vi "HexCenterFinder.vi"() -> ()   [LabVIEW 2019]
uses:
  <vilib>/userDefined/High Color/IMAQdx.ctl
  <vilib>/Analysis/baseanly.llb/Mean (DBL).vi
  <vilib>/vision/driver/NI_Vision_Acquisition_Software.lvlib
  <vilib>/Analysis/NI_AALPro.lvlib
  <vilib>/vision/NI_Vision_Development_Module.lvlib
  <vilib>/Analysis/NI_AALBase.lvlib
panel:
  in  "Component":enum16{"Baseplate", "PCB", "Sensor"}(ring)
  out "concatenated string":string
  out "AngleAvg(3sides)":dbl
  out "CircleBad":T1 {"Radius" format="%.2f"; "Center"."Y" format="%.2f"; "Center"."X" format="%.2f"}
  out "Circle0":T1 {"Radius" format="%.2f"; "Center"."Y" format="%.4f"; "Center"."X" format="%.4f"}
  out "Y 3":dbl
  out "X 3":dbl
  out "Array":dbl[][](array[numeric])
  out "meanY":dbl format="%0.3f"
  out "meanX":dbl format="%0.3f"
  out "Center5":cluster{"X":sgl, "Y":sgl} {"Y" format="%.2f"; "X" format="%.2f"}
  out "Center4":cluster{"X":sgl, "Y":sgl} {"Y" format="%.2f"; "X" format="%.2f"}
  out "Center3":cluster{"X":sgl, "Y":sgl} {"Y" format="%.2f"; "X" format="%.2f"}
  out "Center2":cluster{"X":sgl, "Y":sgl} {"Y" format="%.2f"; "X" format="%.2f"}
  out "Center1":cluster{"X":sgl, "Y":sgl} {"Y" format="%.2f"; "X" format="%.2f"}
  out "Center (3sides)":cluster{"X":sgl, "Y":sgl} {"Y" format="%.4f"; "X" format="%.4f"}
  out "2sides \nBisecting Line":T2 {"Point 2"."Y" format="%.2f"; "Point 2"."X" format="%.2f"; "Point 1"."Y" format="%.2f"; "Point 1"."X" format="%.2f"}
  out "Y 2":dbl
  out "X 2":dbl
  out "Y":dbl
  out "X":dbl
  in  "Ysides":dbl[](array[numeric])=[893.5593, 821.0074, 821.9544]
  in  "Zpos":dbl[](array[numeric])=[66.4386, 66.953, 66.7995, 66.9366, 66.95, 66.95]
  in  "Xsides":dbl[](array[numeric])=[286.53, 329.344, 411.6833, 453.028, 411.403, 328.577]
  in  "Sides to use":enum16{"2 sides", "3 sides", "6 sides"}(ring)=enum."3 sides"
  out "Image":T3(plugin-control)
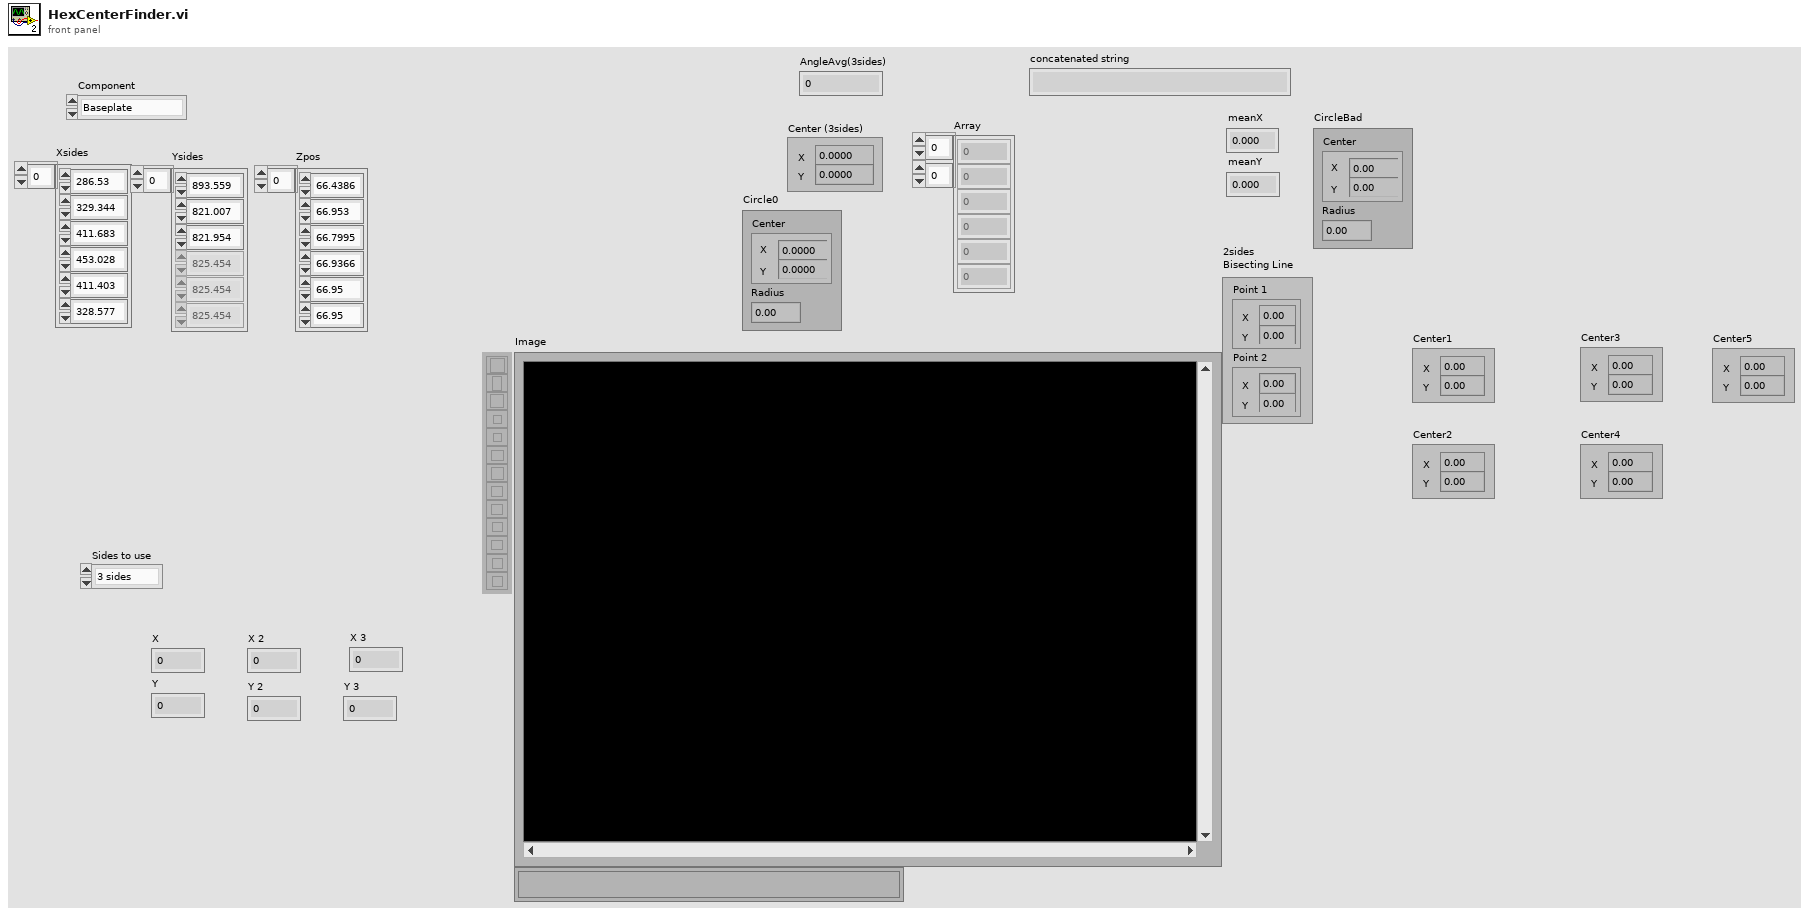
[diagram p1: front panel]
types:
  T1 = cluster{"Center":cluster{"X":sgl, "Y":sgl}, "Radius":dbl}
  T2 = cluster{"Point 1":cluster{"X":sgl, "Y":sgl}, "Point 2":cluster{"X":sgl, "Y":sgl}}
  T3 = typedef "IMAQ Image.ctl" = refnum<image>
  T4 = typedef "Image Type" = u32
  T5 = typedef "IMAQdx.ctl" = refnum<k21>
  T6 = typedef "IMAQ Line" = cluster{"Start X":i32, "Start Y":i32, "End X":i32, "End Y":i32}
  T7 = enum16{"open", "replace", "create", "open or create", "replace or create", "replace or create with confirmation"}
  T8 = cluster{cluster{"X":dbl, "Y":dbl}, cluster{"X":dbl, "Y":dbl}, cluster{"X":dbl, "Y":dbl}}
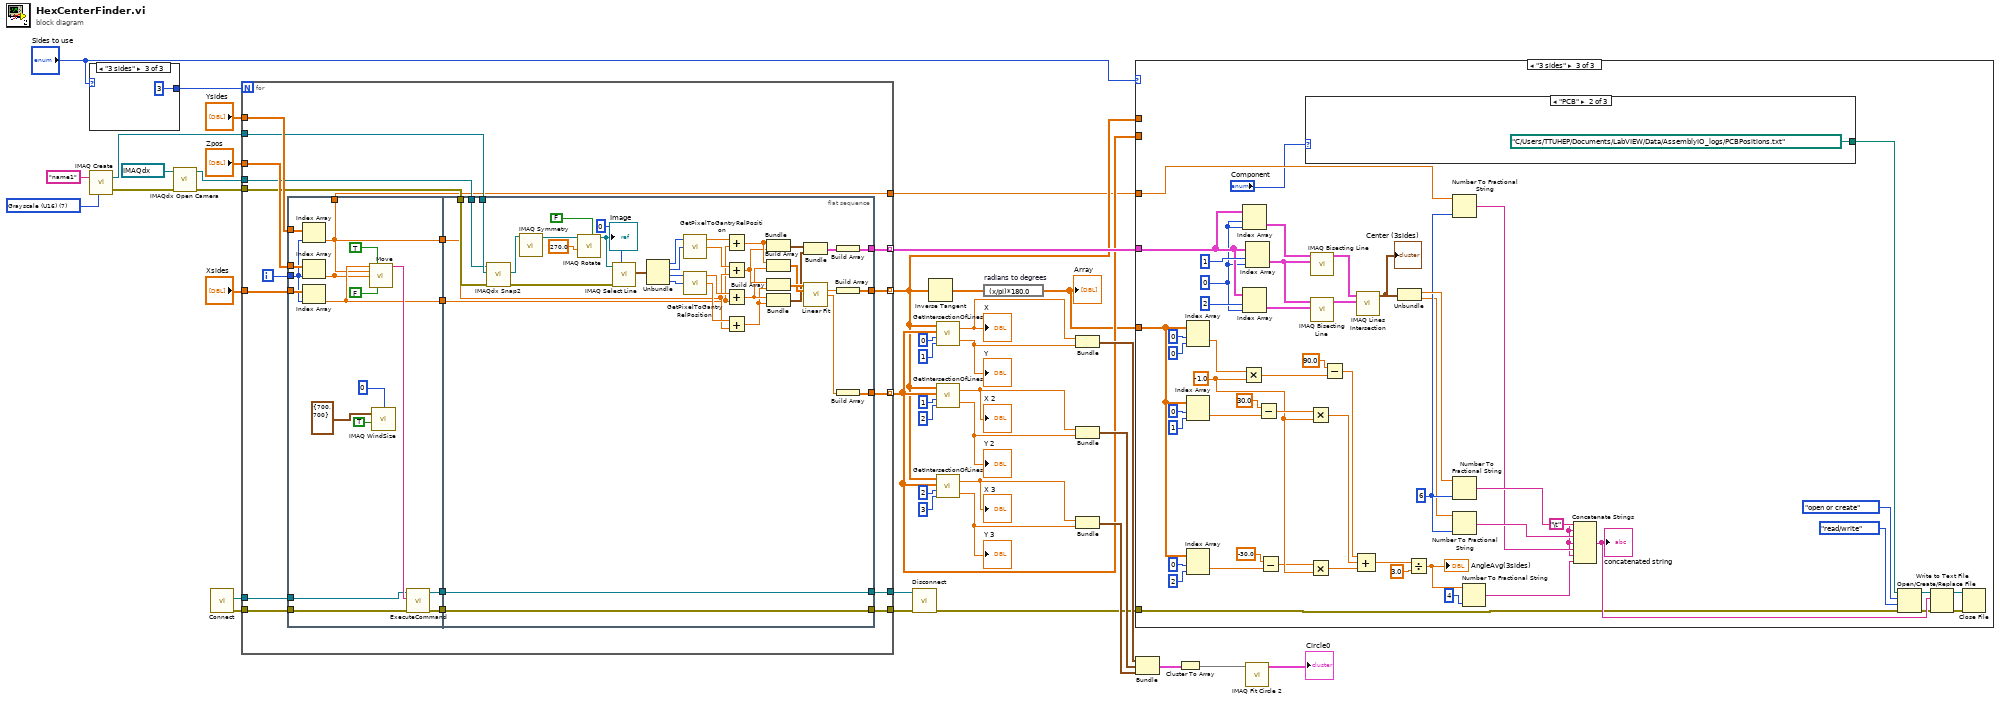
[diagram p0: block diagram]
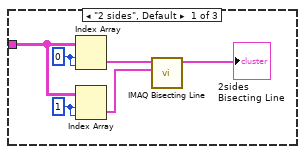
[diagram p2: hidden frame]
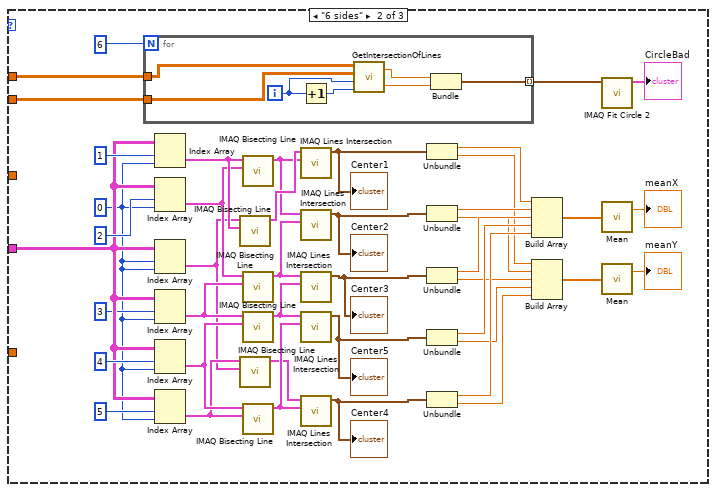
[diagram p3: hidden frame]
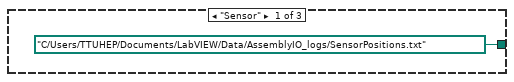
[diagram p4: hidden frame]
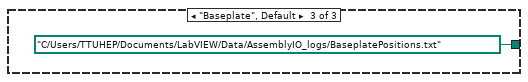
[diagram p5: hidden frame]
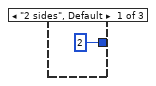
[diagram p6: hidden frame]
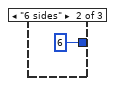
[diagram p7: hidden frame]
diagram:
  w38 = T4 7 items=["Grayscale (U8)", "Grayscale (I16)", "Grayscale (SGL)", "Complex (CSG)", "RGB (U32)", "HSL (U32)", "RGB (U64)", "Grayscale (U16)"] ("Image Type")
  n1 = case shown="\"3 sides\"" "Sides to use" {
    tunnel: [2 6 3] -> w37
    frame "2 sides", Default {
    }
    frame "6 sides" {
    }
    frame "3 sides" {
    }
  }
  n2 = call "IMAQ Create"("Image Name"="name1", "Image Type"=w38) -> ("New Image"=w29:T3, "error out"=w39:errorcluster)  [unwired: 3 in]
  n3 = call <vilib>:"IMAQdx Open Camera.vi"("error in"=w39, "Session In"=T5 "cam0") -> ("error out"=w30:errorcluster, "Session Out"=w28:T5)  [unwired: 8 in]
  n4 = call "Connect.vi"() -> ("error out"=w31:errorcluster, "controller"=w32:refnum<k24>)  [unwired: 10 in]
  n5 = for {
    N: w37 -> [_]
    tunnel: "Xsides" -> [w63]
    tunnel: "Ysides" -> [w62]
    tunnel: "Zpos" -> [w61]
    tunnel: [w59] -> w34
    tunnel: [w58] -> w33
    tunnel: w32 -> [w57]
    tunnel: w31 -> [w56]
    tunnel: w30 -> [w53]
    tunnel: w29 -> [w52]
    tunnel: w28 -> [w51]
    tunnel: [w48] -> w4 mode=indexing
    tunnel: [w47] -> w5 mode=indexing
    tunnel: [w46] -> w21 mode=indexing
    tunnel: [w45] -> w2
    i -> [w60]
    n6 = flat-sequence {
      tunnel: w63 -> [w80]
      tunnel: w62 -> [w79]
      tunnel: w61 -> [w78]
      tunnel: w60 -> [w77]
      tunnel: w57 -> [w71]
      tunnel: w56 -> [w70]
      tunnel: [w73] -> w55
      tunnel: [w72] -> w54
      tunnel: [w69] -> w50
      tunnel: [w68] -> w49
      tunnel: [w67] -> w45
      tunnel: [w116] -> w58
      tunnel: [w117] -> w59
      tunnel: w55 -> [w117]
      tunnel: w54 -> [w116]
      tunnel: w53 -> [w109]
      tunnel: w52 -> [w108]
      tunnel: w51 -> [w107]
      tunnel: w50 -> [w102]
      tunnel: w49 -> [w103]
      tunnel: [w100] -> w48
      tunnel: [w98] -> w47
      tunnel: [w82] -> w46
      frame #0 {
        n7 = Index Array(array=w79, index=w77) -> (element=w68:dbl)
        n8 = Index Array(array=w78, index=w77) -> (element=w67:dbl)
        n9 = Index Array(array=w80, index=w77) -> (element=w69:dbl)
        n10 = call "Move.vi"("X"=w69, "Absolute"=TRUE, "Y"=w68, "Z"=w67, "Move Z first"=FALSE) -> ("Position Gcode"=w74:string)  [unwired: 10 in]
        n11 = call "IMAQ WindSize"("Scrollbars? (N)"=TRUE, "Width & Height"=cluster{"Width":i32, "Height":i32} {"Width"=700, "Height"=700}, "Window Number"=0) -> ()  [unwired: 3 in, 3 out]
        n12 = call "ExecuteCommand.vi"("error in (no error)"=w70, "Command Code"=w74, "controller in"=w71) -> ("error out"=w73:errorcluster, "controller out"=w72:refnum<k24>)  [unwired: 6 in, 1 out]
      }
      frame #1 {
        n13 = call <vilib>:"IMAQdx Snap2.vi"("error in"=w109, "Image In"=w108, "Session In"=w107) -> ("error out"=w110:errorcluster, "Image Out"=w94:T3)  [unwired: 6 in, 1 out]
        n14 = call "IMAQ Symmetry"("Image Src"=w94) -> ("Image Dst Out"=w97:T3)  [unwired: 4 in, 1 out]
        n15 = call "IMAQ Rotate"("Maintain Size"=FALSE, "Angle (degrees)"=sgl 270.0, "Image Src"=w97) -> ("Image Dst Out"=w93:T3)  [unwired: 7 in, 1 out]
        "Image" <- w93
        n16 = call "IMAQ Select Line"("Window Number (0...15)"=0, "error in (no error)"=w110, "Image In"=w93) -> ("Line"=w111:T6)  [unwired: 5 in, 3 out]
        n17 = Unbundle(w111) -> ("Start X"=w112:i32, "Start Y"=w113:i32, "End X"=w114:i32, "End Y"=w115:i32)
        n18 = call "GetPixelToGantryRelPosition.vi"("PixelY"=w113, "PixelX"=w112) -> ("YmmRelGH"=w104:dbl, "XmmRelGH"=w90:dbl)  [unwired: 1 in, 1 out]
        n19 = call "GetPixelToGantryRelPosition.vi"("PixelY"=w115, "PixelX"=w114) -> ("YmmRelGH"=w105:dbl, "XmmRelGH"=w106:dbl)  [unwired: 1 in, 1 out]
        n20 = Add(x=w90, y=w102) -> (x+y=w89:dbl)
        n21 = Add(x=w104, y=w103) -> (x+y=w88:dbl)
        n22 = Add(x=w106, y=w102) -> (x+y=w87:dbl)
        n23 = Add(x=w105, y=w103) -> (x+y=w86:dbl)
        n24 = Bundle(w89, w88) -> (w85:cluster{dbl, dbl})  [unwired: 1 in]
        n25 = Build Array(w89, w87) -> (w91:dbl[])
        n26 = Build Array(w88, w86) -> (w92:dbl[])
        n27 = Bundle(w87, w86) -> (w84:cluster{dbl, dbl})  [unwired: 1 in]
        n28 = Bundle(w85, w84) -> (w83:cluster{cluster{dbl, dbl}, cluster{dbl, dbl}})  [unwired: 1 in]
        n29 = call <vilib>:"Linear Fit.vi"("Y"=w92, "X"=w91) -> ("slope"=w101:dbl, "intercept"=w99:dbl)  [unwired: 9 in, 3 out]
        n30 = Build Array(w83) -> (w82:cluster{cluster{dbl, dbl}, cluster{dbl, dbl}}[])
        n31 = Build Array(w101) -> (w100:dbl[])
        n32 = Build Array(w99) -> (w98:dbl[])
      }
    }
  }
  n33 = call "Disconnect.vi"("error in (no error)"=w34, "controller"=w33) -> ("error out"=w1:errorcluster)  [unwired: 9 in]
  n34 = Inverse Tangent(1:w4) -> (0:w27:dbl[][])
  n35 = call "GetIntersectionOfLines.vi"("Line1Idx"=1, "Line0Idx"=0, "InterceptArray"=w5, "SlopeArray"=w4) -> ("Y"=w16:dbl, "X"=w17:dbl)
  "X" <- w17
  "Y" <- w16
  n36 = call "GetIntersectionOfLines.vi"("Line1Idx"=2, "Line0Idx"=1, "InterceptArray"=w5, "SlopeArray"=w4) -> ("Y"=w14:dbl, "X"=w15:dbl)
  "X 2" <- w15
  "Y 2" <- w14
  n37 = call "GetIntersectionOfLines.vi"("Line1Idx"=3, "Line0Idx"=2, "InterceptArray"=w5, "SlopeArray"=w4) -> ("Y"=w12:dbl, "X"=w13:dbl)
  "X 3" <- w13
  "Y 3" <- w12
  n38 = expression code="(x/pi)*180.0" "radians to degrees"(w27) -> (w3:dbl[][])
  "Array" <- w3
  n39 = Bundle("X"=w17, "Y"=w16) -> (w11:cluster{"X":dbl, "Y":dbl})  [unwired: 1 in]
  n40 = Bundle("X"=w15, "Y"=w14) -> (w10:cluster{"X":dbl, "Y":dbl})  [unwired: 1 in]
  n41 = Bundle("X"=w13, "Y"=w12) -> (w9:cluster{"X":dbl, "Y":dbl})  [unwired: 1 in]
  n42 = case shown="\"3 sides\"" "Sides to use" {
    tunnel: w21 -> [w119 w159 w224]
    tunnel: w5 -> [_ w125 _]
    tunnel: w4 -> [_ w124 _]
    tunnel: w3 -> [_ _ w209]
    tunnel: w2 -> [_ _ w200]
    tunnel: w1 -> [_ _ w179]
    frame "2 sides", Default {
      w121 = 1 ("index (row)")
      w122 = 0 ("index (row)")
      n43 = Index Array(array=w119, index (row)=w122, index (col)=w122) -> (element=w123:cluster{cluster{dbl, dbl}, cluster{dbl, dbl}})
      n44 = Index Array(array=w119, index (row)=w121, index (col)=w121) -> (element=w120:cluster{cluster{dbl, dbl}, cluster{dbl, dbl}})
      n45 = call "IMAQ Bisecting Line"("Line 2"=w120, "Line 1"=w123) -> ("Bisecting Line"=→"2sides \nBisecting Line":T2)  [unwired: 8 in, 1 out]
    }
    frame "6 sides" {
      w148 = 0 ("index (row)")
      n46 = for {
        N: 6 -> [_]
        tunnel: w125 -> [w173]
        tunnel: w124 -> [w172]
        tunnel: [w167] -> w127 mode=indexing
        i -> [w170]
        n47 = Increment(x=w170) -> (x+1=w171:i32)
        n48 = call "GetIntersectionOfLines.vi"("Line1Idx"=w171, "Line0Idx"=w170, "InterceptArray"=w173, "SlopeArray"=w172) -> ("Y"=w168:dbl, "X"=w169:dbl)
        n49 = Bundle("X"=w169, "Y"=w168) -> (w167:cluster{"X":dbl, "Y":dbl})  [unwired: 1 in]
      }
      n50 = Index Array(array=w159, index (row)=1, index (col)=w148) -> (element=w164:cluster{cluster{dbl, dbl}, cluster{dbl, dbl}})
      n51 = Index Array(array=w159, index (row)=2, index (col)=w148) -> (element=w157:cluster{cluster{dbl, dbl}, cluster{dbl, dbl}})
      n52 = Index Array(array=w159, index (row)=w148, index (col)=w148) -> (element=w152:cluster{cluster{dbl, dbl}, cluster{dbl, dbl}})
      n53 = Index Array(array=w159, index (row)=3 ("disabled index (row)"), index (col)=w148) -> (element=w156:cluster{cluster{dbl, dbl}, cluster{dbl, dbl}})
      n54 = Index Array(array=w159, index (row)=4, index (col)=w148) -> (element=w160:cluster{cluster{dbl, dbl}, cluster{dbl, dbl}})
      n55 = Index Array(array=w159, index (row)=5, index (col)=w148) -> (element=w153:cluster{cluster{dbl, dbl}, cluster{dbl, dbl}})
      n56 = call "IMAQ Bisecting Line"("Line 2"=w164, "Line 1"=w152) -> ("Bisecting Line"=w163:T2)  [unwired: 8 in, 1 out]
      n57 = call "IMAQ Bisecting Line"("Line 2"=w152, "Line 1"=w153) -> ("Bisecting Line"=w149:T2)  [unwired: 8 in, 1 out]
      n58 = call "IMAQ Bisecting Line"("Line 2"=w157, "Line 1"=w164) -> ("Bisecting Line"=w155:T2)  [unwired: 8 in, 1 out]
      n59 = call "IMAQ Bisecting Line"("Line 2"=w156, "Line 1"=w157) -> ("Bisecting Line"=w154:T2)  [unwired: 8 in, 1 out]
      n60 = call "IMAQ Bisecting Line"("Line 2"=w160, "Line 1"=w156) -> ("Bisecting Line"=w150:T2)  [unwired: 8 in, 1 out]
      n61 = call "IMAQ Bisecting Line"("Line 2"=w153, "Line 1"=w160) -> ("Bisecting Line"=w151:T2)  [unwired: 8 in, 1 out]
      n62 = call "IMAQ Lines Intersection"("Line 2"=w155, "Line 1"=w163) -> ("Intersection Point"=w147:cluster{"X":sgl, "Y":sgl})  [unwired: 7 in, 2 out]
      "Center1" <- w147
      n63 = call "IMAQ Lines Intersection"("Line 2"=w154, "Line 1"=w155) -> ("Intersection Point"=w145:cluster{"X":sgl, "Y":sgl})  [unwired: 7 in, 2 out]
      "Center2" <- w145
      n64 = call "IMAQ Lines Intersection"("Line 2"=w150, "Line 1"=w154) -> ("Intersection Point"=w144:cluster{"X":sgl, "Y":sgl})  [unwired: 7 in, 2 out]
      "Center3" <- w144
      n65 = call "IMAQ Lines Intersection"("Line 2"=w151, "Line 1"=w150) -> ("Intersection Point"=w143:cluster{"X":sgl, "Y":sgl})  [unwired: 7 in, 2 out]
      "Center5" <- w143
      n66 = call "IMAQ Lines Intersection"("Line 2"=w151, "Line 1"=w149) -> ("Intersection Point"=w142:cluster{"X":sgl, "Y":sgl})  [unwired: 7 in, 2 out]
      "Center4" <- w142
      n67 = Unbundle(w147) -> ("X"=w146:sgl, "Y"=w137:sgl)
      n68 = Unbundle(w145) -> ("X"=w141:sgl, "Y"=w136:sgl)
      n69 = Unbundle(w144) -> ("X"=w140:sgl, "Y"=w135:sgl)
      n70 = Unbundle(w143) -> ("X"=w139:sgl, "Y"=w134:sgl)
      n71 = Unbundle(w142) -> ("X"=w138:sgl, "Y"=w133:sgl)
      n72 = Build Array(w146, w141, w140, w139, w138) -> (w132:sgl[])
      n73 = Build Array(w137, w136, w135, w134, w133) -> (w131:sgl[])
      n74 = call "IMAQ Fit Circle 2"("Radial Points"=w127) -> ("Circle"=→"CircleBad":T1)  [unwired: 5 in, 5 out]
      n75 = call-poly <vilib>:"Mean.vi"("X"=w132) -> ("mean"=→"meanX":dbl)  [unwired: 1 out]
      n76 = call-poly <vilib>:"Mean.vi"("X"=w131) -> ("mean"=→"meanY":dbl)  [unwired: 1 out]
    }
    frame "3 sides" {
      w187 = -1.0 ("y")
      w195 = "\t"
      w199 = i16 6 ("width (-)")
      w222 = 0 ("index (row)")
      n77 = Index Array(array=w209, index (row)=0, index (col)=0 ("disabled index (col)")) -> (element=w191:dbl)
      n78 = Index Array(array=w209, index (row)=0, index (col)=1 ("disabled index (col)")) -> (element=w207:dbl)
      n79 = Index Array(array=w209, index (row)=0, index (col)=2 ("disabled index (col)")) -> (element=w206:dbl)
      n80 = Multiply(x=w191, y=w187) -> (x*y=w190:dbl)
      n81 = Index Array(array=w224, index (row)=w222, index (col)=w222) -> (element=w226:cluster{cluster{dbl, dbl}, cluster{dbl, dbl}})
      n82 = Index Array(array=w224, index (row)=2, index (col)=w222) -> (element=w221:cluster{cluster{dbl, dbl}, cluster{dbl, dbl}})
      n83 = Index Array(array=w224, index (row)=1, index (col)=w222) -> (element=w220:cluster{cluster{dbl, dbl}, cluster{dbl, dbl}})
      n84 = Subtract(x=30.0, y=w207) -> (x-y=w188:dbl)
      n85 = Subtract(x=-30.0, y=w206) -> (x-y=w186:dbl)
      n86 = case shown="\"PCB\"" "Component" {
        tunnel: [path "C:/Users/TTUHEP/Documents/LabVIEW/Data/AssemblyIO_logs/SensorPositions.txt" ("OutFile") path "C:/Users/TTUHEP/Documents/LabVIEW/Data/AssemblyIO_logs/PCBPositions.txt" ("OutFile") path "C:/Users/TTUHEP/Documents/LabVIEW/Data/AssemblyIO_logs/BaseplatePositions.txt" ("OutFile")] -> w174
        frame "Sensor" {
        }
        frame "PCB" {
        }
        frame "Baseplate", Default {
        }
      }
      n87 = Multiply(x=w188, y=w187) -> (x*y=w189:dbl)
      n88 = Multiply(x=w186, y=w187) -> (x*y=w185:dbl)
      n89 = call "IMAQ Bisecting Line"("Line 2"=w220, "Line 1"=w226) -> ("Bisecting Line"=w219:T2)  [unwired: 8 in, 1 out]
      n90 = call "IMAQ Bisecting Line"("Line 2"=w221, "Line 1"=w220) -> ("Bisecting Line"=w218:T2)  [unwired: 8 in, 1 out]
      n91 = Subtract(x=90.0, y=w190) -> (x-y=w204:dbl)
      n92 = call "IMAQ Lines Intersection"("Line 2"=w218, "Line 1"=w219) -> ("Intersection Point"=w217:cluster{"X":sgl, "Y":sgl})  [unwired: 7 in, 2 out]
      "Center (3sides)" <- w217
      n93 = Compound Arithmetic op=ADD(w204, w189, w185) -> (w203:dbl)
      n94 = Unbundle(w217) -> ("X"=w201:sgl, "Y"=w184:sgl)
      n95 = Divide(x=w203, y=3.0) -> (x/y=w194:dbl)
      "AngleAvg(3sides)" <- w194
      n96 = Number To Fractional String(number=w200, precision (6)=w199) -> (F-format string=w196:string)  [unwired: 2 in]
      n97 = Number To Fractional String(number=w201, precision (6)=w199) -> (F-format string=w198:string)  [unwired: 2 in]
      n98 = Number To Fractional String(number=w184, precision (6)=w199) -> (F-format string=w197:string)  [unwired: 2 in]
      n99 = Number To Fractional String(number=w194, precision (6)=i16 4 ("width (-)")) -> (F-format string=w192:string)  [unwired: 2 in]
      n100 = Concatenate Strings(w198, w195, w197, w195, w196, w195, w192) -> (w183:string)
      "concatenated string" <- w183
      n101 = Open/Create/Replace File(file path (use dialog)=w174, error in=w179, operation (0:open)=T7."open or create", access (0:read/write)=enum16{"read/write", "read-only", "write-only"}."read/write") -> (refnum out=w182:refnum<file>, error out=w178:errorcluster)  [unwired: 2 in, 1 out]
      n102 = Write to Text File(file (use dialog)=w182, text=w183, error in=w178) -> (refnum out=w176:refnum<file>, error out=w177:errorcluster)  [unwired: 1 in, 1 out]
      n103 = Close File(refnum=w176, error in=w177) -> ()  [unwired: 2 out]
    }
  }
  n104 = Bundle(w11, w10, w9) -> (w7:T8)  [unwired: 1 in]
  n105 = Cluster To Array(cluster=w7) -> (array=w8:cluster{"X":dbl, "Y":dbl}[])
  n106 = call "IMAQ Fit Circle 2"("Radial Points"=w8) -> ("Circle"=→"Circle0":T1)  [unwired: 5 in, 5 out]
